vi "GxCntExample.vi"(2 "error in (no error)":errorcluster, 3 "Function":enum16{"Frequency", "Period", "Pulse Width"}(ring), 4 "Slot":i16=7) -> (0 "error out":errorcluster, 1 "Measurement":dbl format="%.4e")   [LabVIEW 2010]
panel:
  in  "Force Measurement Ready":bool
  in  "Channel In":i16(ring) items=["Channel A", "Channel B"]
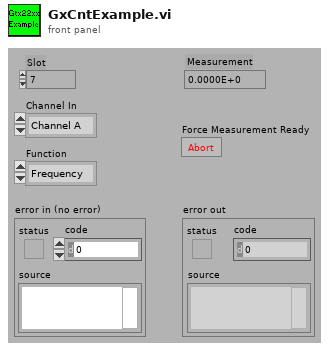
[diagram p1: front panel]
types:
  T1 = enum16{"Trigger Level Fixed", "Trigger Level Auto", "Trigger Level Hold Last"}
  T2 = enum16{"Filter Off", "Filter Auto", "Filter Value Fixed"}
  T3 = enum16{"Arm External", "Arm Off", "Arm Alternate"}
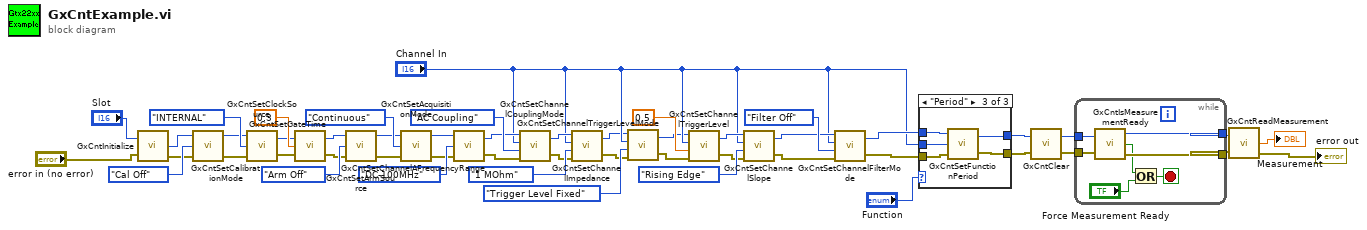
[diagram p0: block diagram]
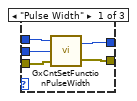
[diagram p2: hidden frame]
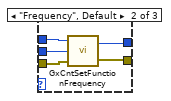
[diagram p3: hidden frame]
diagram:
  n1 = call "GxCntInitialize.vi"("Slot"="Slot", "error in (no error)"="error in (no error)") -> ("Handle"=w23:i16, "error out"=w24:errorcluster)  [unwired: 1 out]
  n2 = call "GxCntSetCalibrationMode.vi"("error in (no error)"=w24, "Mode"=enum16{"Cal Off", "Cal Continuous", "Cal Once"}."Cal Off", "Handle"=w23) -> ("error out"=w21:errorcluster, "Handle copy"=w22:i16)
  n3 = call "GxCntSetClockSource.vi"("error in (no error)"=w21, "Source"=enum16{"INTERNAL", "EXTERNAL", "ALTERNATE"}."INTERNAL", "Handle"=w22) -> ("error out"=w43:errorcluster, "Handle copy"=w42:i16)
  n4 = call "GxCntSetGateTime.vi"("error in (no error)"=w43, "Seconds"=0.3, "Handle"=w42) -> ("error out"=w25:errorcluster, "Handle copy"=w26:i16)
  n5 = call "GxCntSetArmSource.vi"("error in (no error)"=w25, "Source"=T3."Arm Off", "Handle"=w26) -> ("error out"=w19:errorcluster, "Handle copy"=w20:i16)
  n6 = call "GxCntSetAcquisitionMode.vi"("error in (no error)"=w19, "Mode"=enum16{"Continuous", "Single", "Paced"}."Continuous", "Handle"=w20) -> ("error out"=w17:errorcluster, "Handle copy"=w18:i16)
  n7 = call "GxCntSetChannelAFrequencyRange.vi"("error in (no error)"=w17, "Range"=enum16{"DC-100MHz", "DC-1.3GHz"}."DC-100MHz", "Handle"=w18) -> ("error out"=w15:errorcluster, "Handle copy"=w16:i16)
  n8 = call "GxCntSetChannelCouplingMode.vi"("error in (no error)"=w15, "Mode"=enum16{"AC Coupling", "DC Coupling"}."AC Coupling", "Channel"="Channel In", "Handle"=w16) -> ("error out"=w14:errorcluster, "Handle copy"=w13:i16)
  n9 = call "GxCntSetChannelImpedance.vi"("error in (no error)"=w14, "Mode"=enum16{"1 MOhm", "50 Ohm"}."1 MOhm", "Channel"="Channel In", "Handle"=w13) -> ("error out"=w3:errorcluster, "Handle copy"=w4:i16)
  n10 = call "GxCntSetChannelTriggerLevelMode.vi"("error in (no error)"=w3, "Mode"=T1."Trigger Level Fixed", "Channel"="Channel In", "Handle"=w4) -> ("error out"=w1:errorcluster, "Handle copy"=w2:i16)
  n11 = call "GxCntSetChannelTriggerLevel.vi"("error in (no error)"=w1, "Voltage"=0.5, "Channel"="Channel In", "Handle"=w2) -> ("error out"=w12:errorcluster, "Handle copy"=w11:i16)
  n12 = call "GxCntSetChannelSlope.vi"("error in (no error)"=w12, "Slope"=enum16{"Rising Edge", "Falling Edge"}."Rising Edge", "Channel"="Channel In", "Handle"=w11) -> ("error out"=w9:errorcluster, "Handle copy"=w10:i16)
  n13 = call "GxCntSetChannelFilterMode.vi"("error in (no error)"=w9, "Mode"=T2."Filter Off", "Channel"="Channel In", "Handle"=w10) -> ("error out"=w7:errorcluster, "Handle copy"=w8:i16)
  n14 = case shown="\"Period\"" "Function" {
    tunnel: w8 -> [w55 w60 w65]
    tunnel: [w54 w59 w64] -> w39
    tunnel: w7 -> [w53 w58 w63]
    tunnel: [w52 w57 w62] -> w38
    tunnel: "Channel In" -> [w51 w56 w61]
    frame "Pulse Width" {
      n15 = call "GxCntSetFunctionPulseWidth.vi"("error in (no error)"=w53, "Channel"=w51, "Handle"=w55) -> ("error out"=w52:errorcluster, "Handle copy"=w54:i16)
    }
    frame "Frequency", Default {
      n16 = call "GxCntSetFunctionFrequency.vi"("error in (no error)"=w58, "Channel"=w56, "Handle"=w60) -> ("error out"=w57:errorcluster, "Handle copy"=w59:i16)
    }
    frame "Period" {
      n17 = call "GxCntSetFunctionPeriod.vi"("error in (no error)"=w63, "Channel"=w61, "Handle"=w65) -> ("error out"=w62:errorcluster, "Handle copy"=w64:i16)
    }
  }
  n18 = call "GxCntClear.vi"("error in (no error)"=w38, "Handle"=w39) -> ("error out"=w36:errorcluster, "Handle Out"=w37:i16)
  n19 = while {
    tunnel: w37 -> [w72]
    tunnel: w36 -> [w71]
    tunnel: [w70] -> w41
    tunnel: [w69] -> w40
    stop <- w68 stop-if-true
    n20 = call "GxCntIsMeasurementReady.vi"("Handle"=w72, "error in (no error)"=w71) -> ("Handle copy"=w70:i16, "Ready"=w67:bool, "error out"=w69:errorcluster)
    n21 = Or(x=w67, y="Force Measurement Ready") -> (x .or. y?=w68:bool)
  }
  n22 = call "GxCntReadMeasurement.vi"("Handle"=w41, "error in (no error)"=w40) -> ("Measurement"=→"Measurement":dbl, "error out"=→"error out":errorcluster)  [unwired: 1 out]
